vi "TDC_Prototype.vi"() -> ()   [LabVIEW 2025]
uses:
  Desktop/STM-Auto-Project/QMH CTLS/Scan_Params (QMH).ctl
  TDC_SubVI/TEMP_SWEEPER.ctl
  Downloads/OneDrive_2025-09-03/Instrument Controls/Temp Cntrl.ctl
  Desktop/Magnetic Drift Correction/XY_Coords(Final).ctl
panel:
  out "Z-Controller on/off status":bool
  in  "Field and Temp Range":T1={"VISA (Magnet)"="COM4", "Fields(T)"=[], "Temps(K)"=[], "VISA (Temp) "="COM1"}
  out "error out":errorcluster
  in  "Serial Configuration":T2={"Baud Rate"=57600, "Parity"=1, "Data Bits"=7, "Stop Bits"=10, "Flow Control"=0}
  out "Current Index":i32
  out "Translation (m)":T3
  out "Final coordinates (m)":cluster{"Xc":sgl, "Yc":sgl} {"Yc" format="%.4p"; "Xc" format="%.4p"}
  out "Initial coordinates (m)":cluster{"Xc":sgl, "Yc":sgl} {"Yc" format="%.4p"; "Xc" format="%.4p"}
  in  "stop":bool
  in  "Start":bool
  # "Main goals,\n\nSet base line: Do initial bias and scan\n\nChange temp: Init temp, temp on, temp stab,\n\nInter scan, move frame, final scan, bias shit,\n\nNext temp? Prep next field though reinialization, determine if higher range is needed, apply field by changing setpoint\n\nInter scan, move frame, final scan, bias shit,"
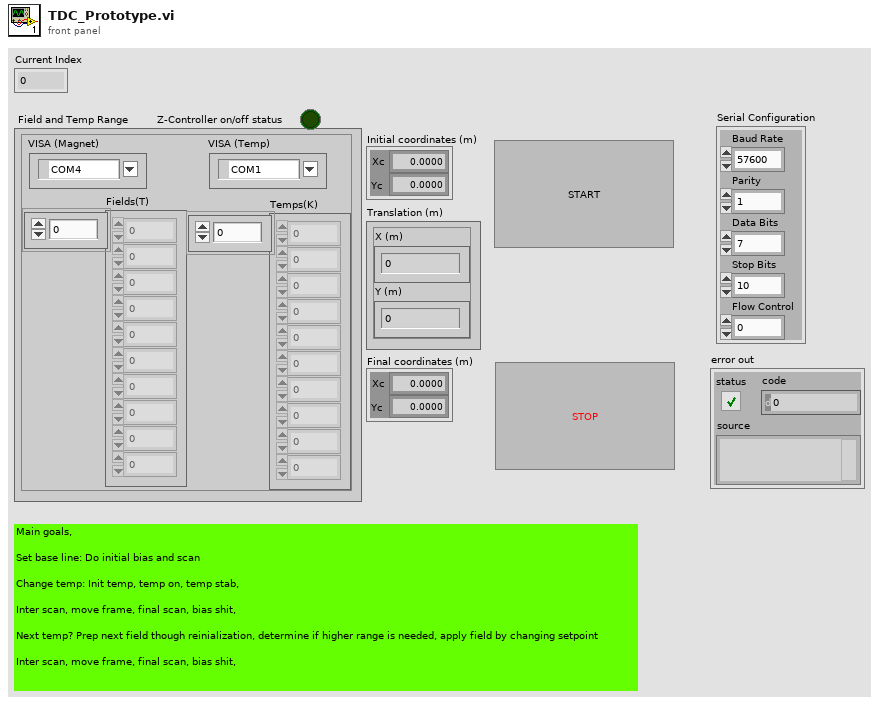
[diagram p1: front panel]
types:
  T1 = cluster{"VISA (Magnet)":refnum<visa-resource-name>, "Fields(T)":dbl[], "Temps(K)":dbl[], "VISA (Temp) ":refnum<visa-resource-name>}
  T2 = cluster{"Baud Rate":u32, "Parity":u16, "Data Bits":u16, "Stop Bits":u16, "Flow Control":u16}
  T3 = typedef "XY_Coords(Final).ctl" = cluster{"X (m)":dbl, "Y (m)":dbl}
  T4 = enum16{"1. BIAS", "2. INIT_SCAN", "3. SCAN_IDLE", "4. INTER_SCAN", "5. NEW_COORDS_&_FRAME", "6. FINAL_SCAN", "7. POLL BIAS ", "8. Z-CONT.", "9. STOP"}
  T5 = enum16{"SET TEMP", "SWEEP IDLE", "NEXT TEMP", "SWEEP DONE"}
  T6 = enum16{"1. INIT TEMP", "2. TC ON", "3. POLL_TEMPS", "4. TEMP_STAB", "5. TC IDLE", "6. APPLY NEXT TEMP", "7. TC OFF (Reset)"}
  T7 = typedef "Temp Cntrl.ctl" = cluster{"Range (0:Off)":u16, "Manual Output (0.00 %)":dbl, "Rate (D) (0.0 %)":dbl, "Reset (I) (20.0)":dbl, "Gain (P) (50.0)":dbl, "Power Up Enable (F: Disable)":bool, "Max User Current (2.000)":dbl, "Heater Resistance (1:25 Ohms)":u16, "Max Current (0:User Specified)":u16, "Heater Out Display (1:Current)":u16, "Mode (0:Off)":u16, "Input (0:None)":u16, "Target Temp (K)":dbl, "Serial Configuration":cluster{"Baud Rate":u32, "Parity":u16, "Data Bits":u16, "Stop Bits":u16, "Flow Control":u16}, "VISA resource name":refnum<visa-resource-name>, "Configure Control Parameters (0: Configure)":u16, "Enable Setpoint (F:Disable)":bool, "Input (0:A)":u16, "Data Source (0:Kelvin)":u16, "Output's Control Loop (1:1)":u16, "STND DEV Threshold ":dbl, "Mean Tolerance ":dbl, "Current State":enum16{"1. INIT TEMP", "2. TC ON", "3. POLL_TEMPS", "4. TEMP_STAB", "5. TC IDLE", "6. APPLY NEXT TEMP", "7. TC OFF (Reset)"}}
  T8 = typedef "TEMP_SWEEPER.ctl" = cluster{"Temps(K)":dbl[], "Sweep States":enum16{"SET TEMP", "SWEEP IDLE", "NEXT TEMP", "SWEEP DONE"}}
  T9 = typedef "Scan_Params (QMH).ctl" = cluster{"Setpoint (I)":dbl[], "Bias (V)":dbl[], "Number of scans":u8, "Port number (3364)":u32, "Avoid zero threshold (V)":dbl, "Current State":enum16{"1. BIAS", "2. INIT_SCAN", "3. SCAN_IDLE", "4. INTER_SCAN", "5. NEW_COORDS_&_FRAME", "6. FINAL_SCAN", "7. POLL BIAS ", "8. Z-CONT.", "9. STOP"}}
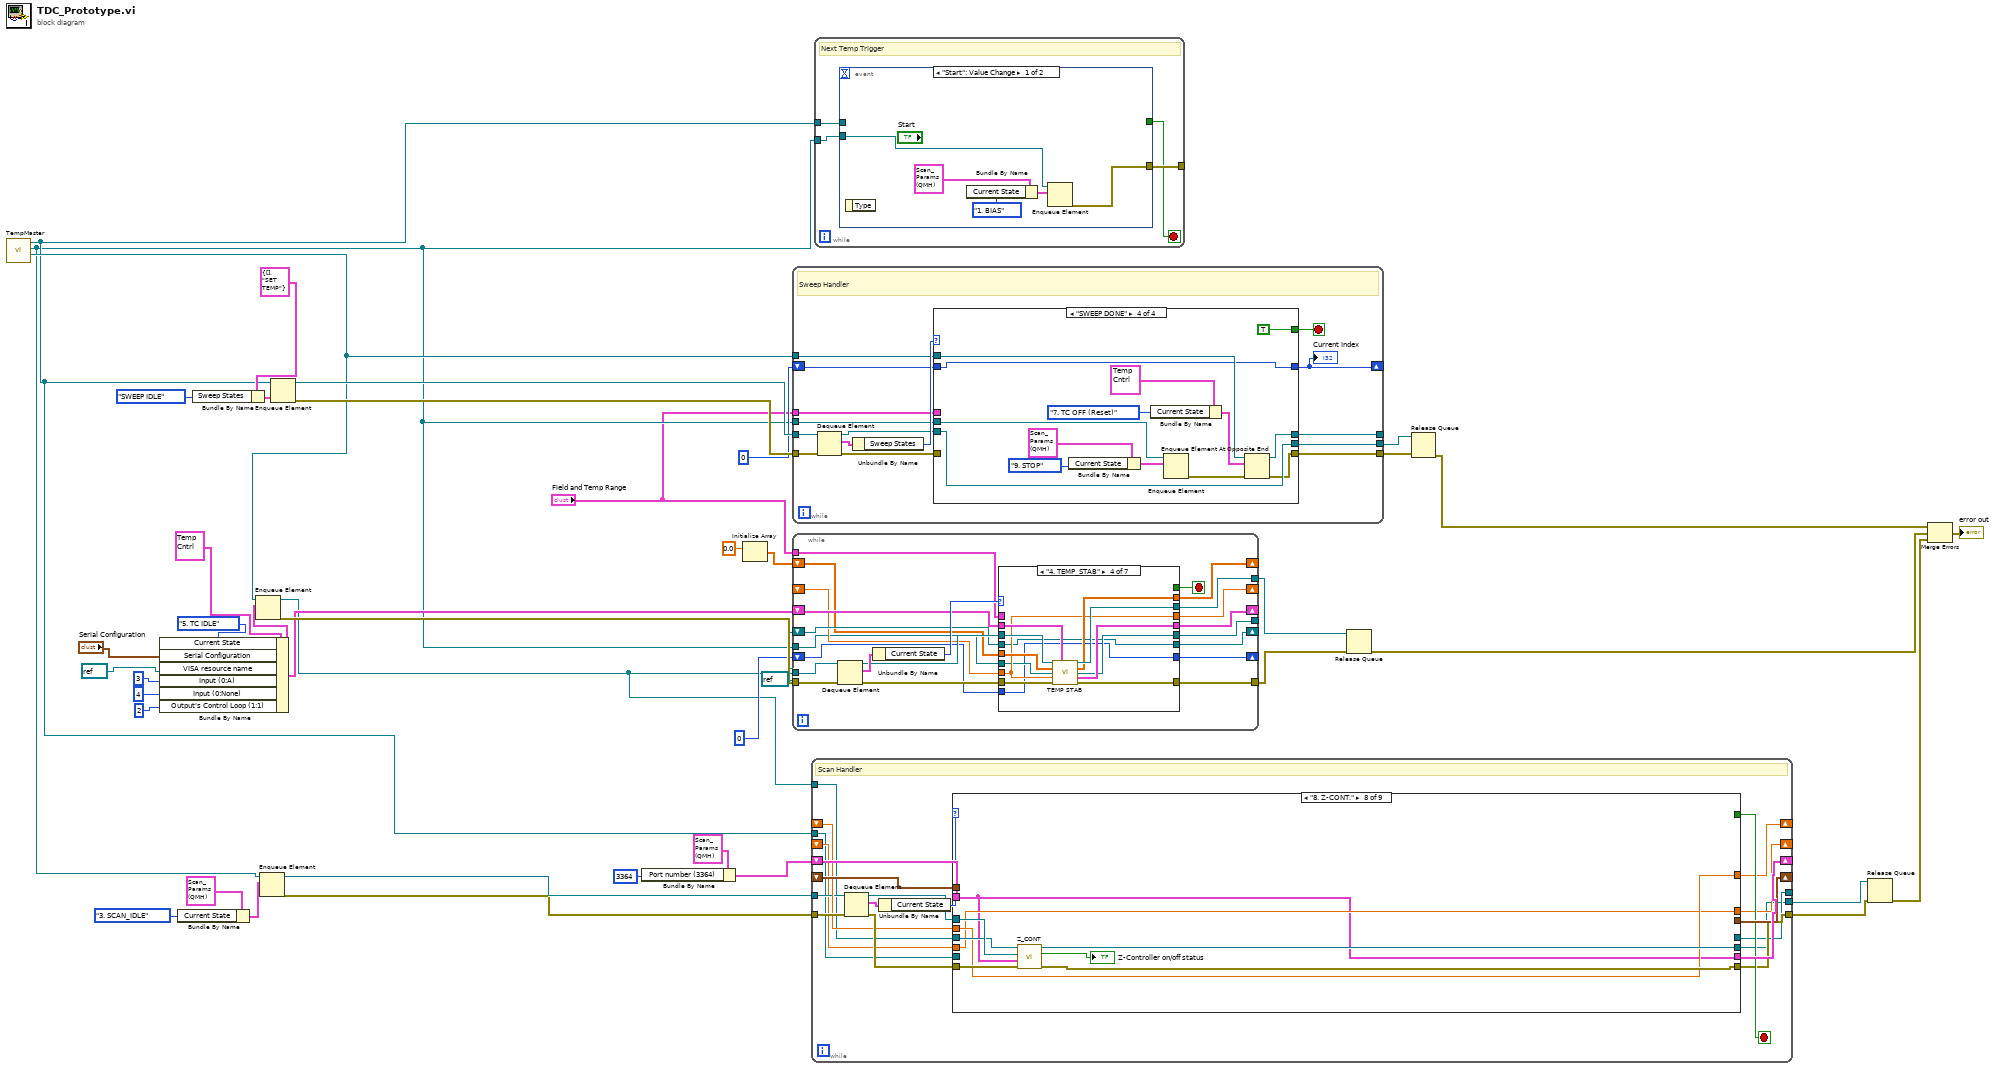
[diagram p0: block diagram]
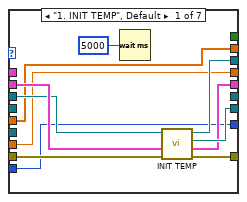
[diagram p2: hidden frame]
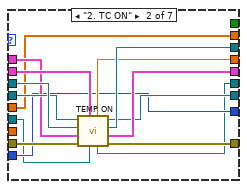
[diagram p3: hidden frame]
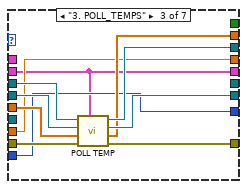
[diagram p4: hidden frame]
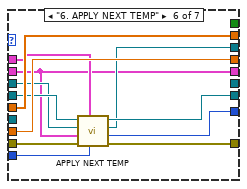
[diagram p6: hidden frame]
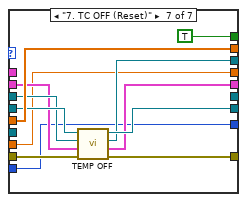
[diagram p7: hidden frame]
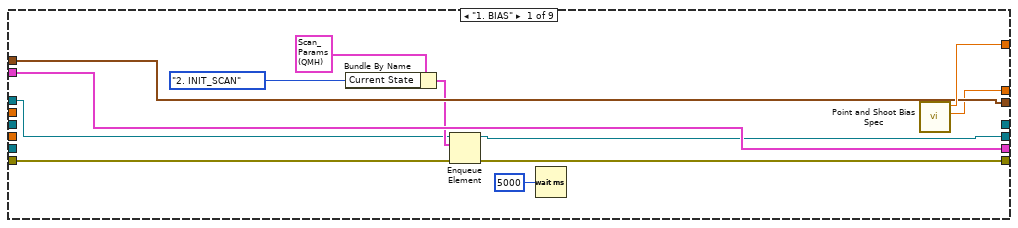
[diagram p8: hidden frame]
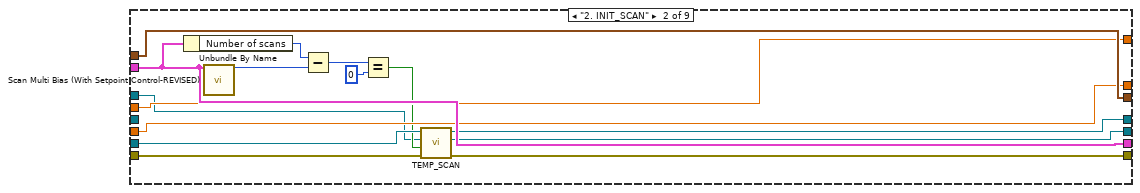
[diagram p9: hidden frame]
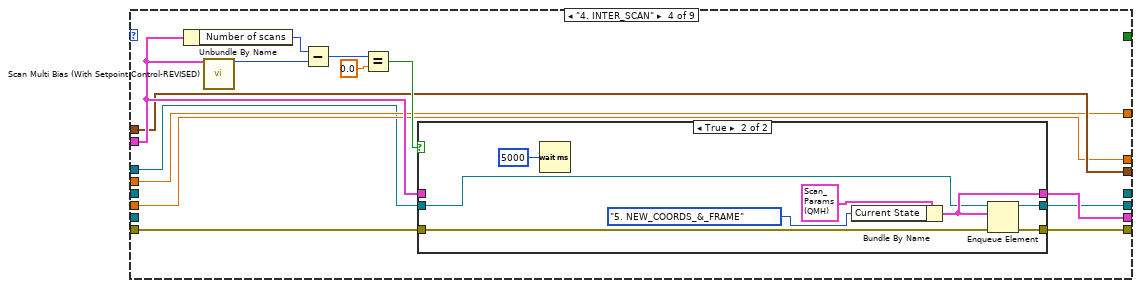
[diagram p11: hidden frame]
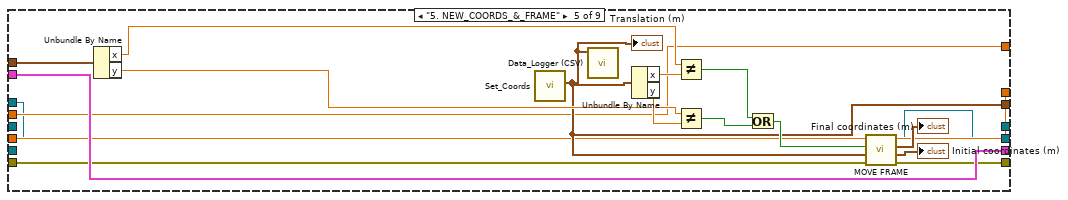
[diagram p13: hidden frame]
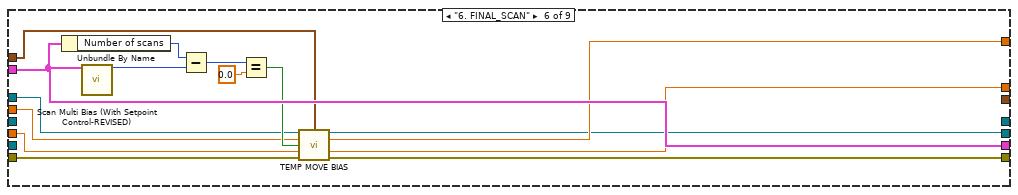
[diagram p14: hidden frame]
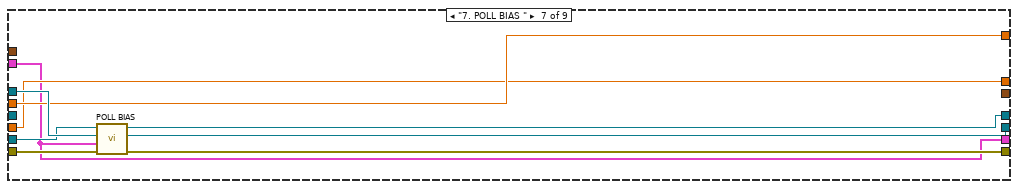
[diagram p15: hidden frame]
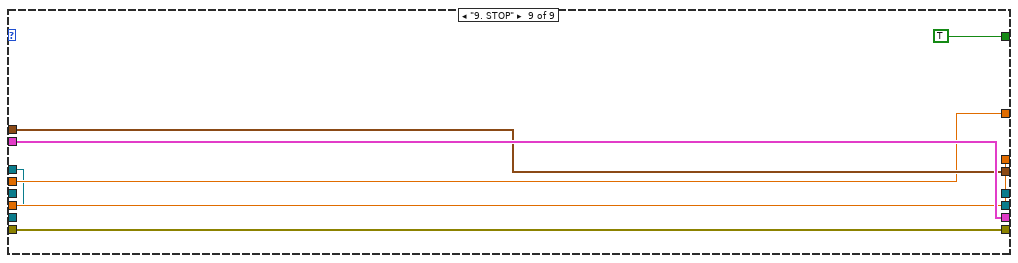
[diagram p16: hidden frame]
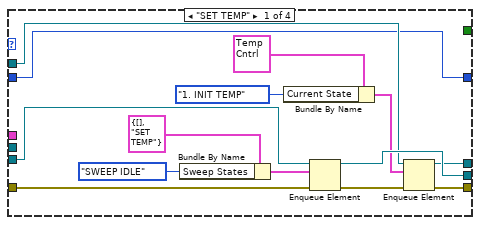
[diagram p17: hidden frame]
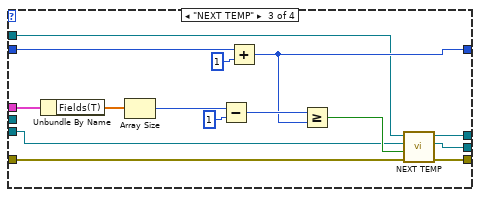
[diagram p19: hidden frame]
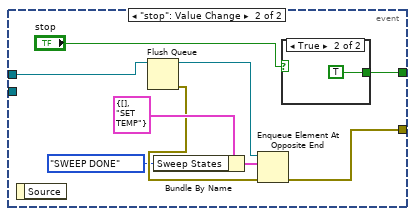
[diagram p20: hidden frame]
diagram:
  n1 = call "TempMaster.vi"() -> ("TempQ"=w27:refnum<queue>, "ScanQ"=w12:refnum<queue>, "SweepQ"=w17:refnum<queue>)  [unwired: 9 in]
  n2 = Bundle By Name(cluster=T7 {"Range (0:Off)"=0, "Manual Output (0.00 %)"=0.0, "Rate (D) (0.0 %)"=0.0, "Reset (I) (20.0)"=20.0, "Gain (P) (50.0)"=50.0, "Power Up Enable (F: Disable)"=FALSE, "Max User Current (2.000)"=2.0, "Heater Resistance (1:25 Ohms)"=1, "Max Current (0:User Specified)"=0, "Heater Out Display (1:Current)"=1, "Mode (0:Off)"=1, "Input (0:None)"=4, "Target Temp (K)"=5.0, "Serial Configuration"={"Baud Rate"=57600, "Parity"=1, "Data Bits"=7, "Stop Bits"=10, "Flow Control"=0}, "VISA resource name"="", "Configure Control Parameters (0: Configure)"=0, "Enable Setpoint (F:Disable)"=FALSE, "Input (0:A)"=3, "Data Source (0:Kelvin)"=0, "Output's Control Loop (1:1)"=2, "STND DEV Threshold "=0.1, "Mean Tolerance "=0.02, "Current State"=enum."1. INIT TEMP"} ("element"), "Current State"=T6."5. TC IDLE", "Serial Configuration"="Serial Configuration", "VISA resource name"=refnum<visa-resource-name> refnum, "Input (0:A)"=u16 3, "Input (0:None)"=u16 4, "Output's Control Loop (1:1)"=u16 2) -> (w22:T7)
  n3 = Bundle By Name(cluster=T9 {"Setpoint (I)"=[], "Bias (V)"=[], "Number of scans"=1, "Port number (3364)"=3364, "Avoid zero threshold (V)"=0.004999999888241291, "Current State"=enum."1. BIAS"} ("element"), "Current State"=T4."3. SCAN_IDLE") -> (w37:T9)
  n4 = Bundle By Name(cluster=T8 {"Temps(K)"=[], "Sweep States"=enum."SET TEMP"} ("Temp and Field Range"), "Sweep States"=T5."SWEEP IDLE") -> (w41:T8)
  n5 = Enqueue Element(queue=w27, element=w22) -> (queue out=w1:refnum<queue>, error out=w28:errorcluster)  [unwired: 2 in, 1 out]
  n6 = Enqueue Element(queue=w12, element=w37) -> (queue out=w39:refnum<queue>, error out=w38:errorcluster)  [unwired: 2 in, 1 out]
  n7 = Enqueue Element(queue=w17, element=w41) -> (queue out=w42:refnum<queue>, error out=w40:errorcluster)  [unwired: 2 in, 1 out]
  n8 = Bundle By Name(cluster=T9 {"Setpoint (I)"=[], "Bias (V)"=[], "Number of scans"=1, "Port number (3364)"=3364, "Avoid zero threshold (V)"=0.004999999888241291, "Current State"=enum."1. BIAS"} ("element"), "Port number (3364)"=u32 3364) -> (w34:T9)
  n9 = Initialize Array(0.0 ("element")) -> (w18:dbl[])  [unwired: 1 in]
  n10 = while {
    tunnel: w42 -> [w57]
    shift-right: [w50] -> _
    shift-left: 0 ("Current Index") -> [w51]
    tunnel: w27 -> [w49]
    tunnel: w40 -> [w56]
    tunnel: "Field and Temp Range" -> [w52]
    tunnel: [w48] -> w9
    tunnel: [w47] -> _
    tunnel: [w46] -> w8
    tunnel: w12 -> [w44]
    stop <- w43 stop-if-true
    # "Sweep Handler"
    n11 = Dequeue Element(queue=w57, error in (no error)=w56) -> (queue out=w53:refnum<queue>, element=w55:T8, error out=w45:errorcluster)  [unwired: 1 in, 1 out]
    n12 = Unbundle By Name(w55) -> ("Sweep States"=w54:T5)
    n13 = case shown="\"SWEEP DONE\"" w54 {
      tunnel: w53 -> [w71 w73 w80 w96]
      tunnel: w52 -> [_ _ w86 _]
      tunnel: w51 -> [w60 w75 w84 w94]
      tunnel: [w60 w75 w83 w94] -> w50
      tunnel: w49 -> [w63 w74 w81 w103]
      tunnel: [w66 w73 w76 w96] -> w48
      tunnel: [w62 w74 w77 w97] -> w47
      tunnel: [w61 w72 w79 w95] -> w46
      tunnel: w45 -> [w68 w72 w78 _]
      tunnel: w44 -> [_ _ _ w101]
      tunnel: [_ _ _ TRUE] -> w43
      frame "SET TEMP" {
        n14 = Bundle By Name(cluster=T8 {"Temps(K)"=[], "Sweep States"=enum."SET TEMP"} ("Temp and Field Range"), "Sweep States"=T5."SWEEP IDLE") -> (w69:T8)
        n15 = Bundle By Name(cluster=T7 {"Range (0:Off)"=0, "Manual Output (0.00 %)"=0.0, "Rate (D) (0.0 %)"=0.0, "Reset (I) (20.0)"=20.0, "Gain (P) (50.0)"=50.0, "Power Up Enable (F: Disable)"=FALSE, "Max User Current (2.000)"=2.0, "Heater Resistance (1:25 Ohms)"=1, "Max Current (0:User Specified)"=0, "Heater Out Display (1:Current)"=1, "Mode (0:Off)"=1, "Input (0:None)"=4, "Target Temp (K)"=5.0, "Serial Configuration"={"Baud Rate"=57600, "Parity"=1, "Data Bits"=7, "Stop Bits"=10, "Flow Control"=0}, "VISA resource name"="", "Configure Control Parameters (0: Configure)"=0, "Enable Setpoint (F:Disable)"=FALSE, "Input (0:A)"=3, "Data Source (0:Kelvin)"=0, "Output's Control Loop (1:1)"=2, "STND DEV Threshold "=0.1, "Mean Tolerance "=0.02, "Current State"=enum."1. INIT TEMP"} ("element"), "Current State"=T6."1. INIT TEMP") -> (w64:T7)
        n16 = Enqueue Element(queue=w71, element=w69, error in (no error)=w68) -> (queue out=w66:refnum<queue>, error out=w67:errorcluster)  [unwired: 1 in, 1 out]
        n17 = Enqueue Element(queue=w63, element=w64, error in (no error)=w67) -> (queue out=w62:refnum<queue>, error out=w61:errorcluster)  [unwired: 1 in, 1 out]
      }
      frame "SWEEP IDLE" {
      }
      frame "NEXT TEMP" {
        n18 = Unbundle By Name(w86) -> ("Fields(T)"=w85:dbl[])
        n19 = Array Size(array=w85) -> (size(s)=w89:i32)
        n20 = Subtract(x=w89, y=1) -> (x-y=w87:i32)
        n21 = Add(x=w84, y=1) -> (x+y=w83:i32)
        n22 = Greater Or Equal?(x=w87, y=w83) -> (x >= y?=w82:bool)
        n23 = call "NEXT TEMP.vi"("error in (no error)"=w78, "Boolean"=w82, "SweepQ"=w80, "TempQ"=w81) -> ("error out"=w79:errorcluster, "SweepQ Out"=w76:refnum<queue>, "TEMPQ Out"=w77:refnum<queue>)  [unwired: 5 in]
      }
      frame "SWEEP DONE" {
        n24 = Bundle By Name(cluster=T9 {"Setpoint (I)"=[], "Bias (V)"=[], "Number of scans"=1, "Port number (3364)"=3364, "Avoid zero threshold (V)"=0.004999999888241291, "Current State"=enum."1. BIAS"} ("element"), "Current State"=T4."9. STOP") -> (w100:T9)
        n25 = Bundle By Name(cluster=T7 {"Range (0:Off)"=0, "Manual Output (0.00 %)"=0.0, "Rate (D) (0.0 %)"=0.0, "Reset (I) (20.0)"=20.0, "Gain (P) (50.0)"=50.0, "Power Up Enable (F: Disable)"=FALSE, "Max User Current (2.000)"=2.0, "Heater Resistance (1:25 Ohms)"=1, "Max Current (0:User Specified)"=0, "Heater Out Display (1:Current)"=1, "Mode (0:Off)"=1, "Input (0:None)"=4, "Target Temp (K)"=5.0, "Serial Configuration"={"Baud Rate"=57600, "Parity"=1, "Data Bits"=7, "Stop Bits"=10, "Flow Control"=0}, "VISA resource name"="", "Configure Control Parameters (0: Configure)"=0, "Enable Setpoint (F:Disable)"=FALSE, "Input (0:A)"=3, "Data Source (0:Kelvin)"=0, "Output's Control Loop (1:1)"=2, "STND DEV Threshold "=0.1, "Mean Tolerance "=0.02, "Current State"=enum."1. INIT TEMP"} ("element"), "Current State"=T6."7. TC OFF (Reset)") -> (w98:T7)
        n26 = Enqueue Element(queue=w101, element=w100) -> (error out=w104:errorcluster)  [unwired: 2 in, 2 out]
        n27 = Enqueue Element At Opposite End(queue=w103, element=w98, error in (no error)=w104) -> (queue out=w97:refnum<queue>, error out=w95:errorcluster)  [unwired: 1 in, 1 out]
      }
    }
    "Current Index" <- w50
  }
  n28 = while {
    tunnel: w1 -> [w126]
    tunnel: w28 -> [w125]
    shift-right: [w115] -> _
    shift-left: w22 -> [w122]
    tunnel: "Field and Temp Range" -> [w120]
    shift-right: [w119] -> _
    shift-left: refnum<visa-resource-name> refnum ("VISA resource name out") -> [w114]
    tunnel: [w118] -> w10
    tunnel: [w116] -> w11
    shift-right: [w110] -> _
    shift-left: _ -> [w113]
    shift-right: [w111] -> _
    shift-left: w18 -> [w112]
    tunnel: w12 -> [w109]
    tunnel: [w108] -> _
    shift-right: [w106] -> _
    shift-left: 0 -> [w107]
    stop <- w105 stop-if-true
    n29 = Dequeue Element(queue=w126, error in (no error)=w125) -> (queue out=w117:refnum<queue>, element=w124:T7, error out=w121:errorcluster)  [unwired: 1 in, 1 out]
    n30 = Unbundle By Name(w124) -> ("Current State"=w123:T6)
    n31 = case shown="\"4. TEMP_STAB\"" w123 {
      tunnel: w122 -> [w137 w151 w152 w173 w177 w183 w201]
      tunnel: w121 -> [w136 w145 w161 w172 w178 w189 w204]
      tunnel: w120 -> [_ w144 _ _ _ w184 _]
      tunnel: [w135 w143 w160 w163 w179 w188 w203] -> w119
      tunnel: [w132 w148 w157 w170 w178 w185 w200] -> w118
      tunnel: w117 -> [w134 w150 w159 w174 w180 w187 w202]
      tunnel: [w133 w149 w158 w171 w180 w186 w199] -> w116
      tunnel: [w130 w147 w152 w167 w177 w183 w198] -> w115
      tunnel: w114 -> [_ w146 w162 w163 w179 w190 w205]
      tunnel: [w128 w142 w154 w168 w181 w193 w196] -> w110
      tunnel: w113 -> [w128 _ w154 w168 w181 w193 w196]
      tunnel: w112 -> [w129 w141 w156 w175 w182 w194 w206]
      tunnel: [w129 w141 w155 w169 w182 w194 w206] -> w111
      tunnel: w109 -> [_ w139 _ w166 _ _ _]
      tunnel: [_ w138 _ w165 _ _ _] -> w108
      tunnel: w107 -> [w127 w140 w153 w164 w176 w192 w197]
      tunnel: [w127 w140 w153 w164 w176 w191 w197] -> w106
      tunnel: [_ _ _ _ _ _ TRUE] -> w105
      frame "1. INIT TEMP", Default {
        n32 = Wait (ms)(milliseconds to wait=u32 5000) -> ()  [unwired: 1 out]
        n33 = call "INIT TEMP.vi"("error in (no error)"=w136, "element"=w137, "Queue in"=w134) -> ("error out"=w132:errorcluster, "output cluster"=w130:T7, "VISA resource name out"=w135:refnum<visa-resource-name>, "Queue out"=w133:refnum<queue>)  [unwired: 5 in]
      }
      frame "2. TC ON" {
        n34 = call "TEMP ON.vi"("ScanQ in"=w139, "element in"=w151, "error in (no error)"=w145, "Field and Temp Range"=w144, "TempQ in"=w150, "VISA Refnum in"=w146) -> ("error out"=w148:errorcluster, "element out"=w147:T7, "TempQ out"=w149:refnum<queue>, "VISA Refnum out"=w143:refnum<visa-resource-name>, "ScanQ out"=w138:refnum<queue>, "Setpoint"=w142:dbl)
      }
      frame "3. POLL_TEMPS" {
        n35 = call "POLL TEMP.vi"("element"=w152, "error in (no error)"=w161, "Array in"=w156, "VISA resource name in"=w162, "Queue in"=w159) -> ("error out"=w157:errorcluster, "Array"=w155:dbl[], "VISA resource name out"=w160:refnum<visa-resource-name>, "Queue out"=w158:refnum<queue>)  [unwired: 3 in]
      }
      frame "4. TEMP_STAB" {
        n36 = call "TEMP STAB.vi"("Queue in"=w174, "element in"=w173, "Array in"=w175, "ScanQ In"=w166, "Setpoint"=w168, "error in (no error)"=w172) -> ("Queue out"=w171:refnum<queue>, "Array out"=w169:dbl[], "ScanQ"=w165:refnum<queue>, "element out"=w167:T7, "error out"=w170:errorcluster)  [unwired: 5 in]
      }
      frame "5. TC IDLE" {
      }
      frame "6. APPLY NEXT TEMP" {
        n37 = call "APPLY NEXT TEMP.vi"("Numeric in"=w192, "Field and Temp Range"=w184, "error in (no error)"=w189, "element in"=w183, "TempQ in"=w187, "VISA Refnum in"=w190) -> ("error out"=w185:errorcluster, "Numeric out"=w191:i32, "TempQ out"=w186:refnum<queue>, "VISA Refnum out"=w188:refnum<visa-resource-name>)  [unwired: 2 in]
      }
      frame "7. TC OFF (Reset)" {
        n38 = call "TEMP OFF.vi"("error in (no error)"=w204, "element in"=w201, "TempQ in"=w202, "VISA Refnum in"=w205) -> ("error out"=w200:errorcluster, "element out"=w198:T7, "TempQ out"=w199:refnum<queue>, "VISA Refnum out"=w203:refnum<visa-resource-name>)  [unwired: 4 in]
      }
    }
  }
  n39 = while {
    tunnel: w38 -> [w220]
    shift-right: [w225] -> _
    shift-left: w34 -> [w226]
    shift-right: [w224] -> _
    shift-left: _ -> [w223]
    tunnel: [w221] -> w36
    tunnel: [w218] -> _
    shift-right: [w216] -> _
    shift-left: _ -> [w217]
    tunnel: w39 -> [w215]
    shift-right: [w212] -> _
    shift-left: _ -> [w211]
    tunnel: w17 -> [w210]
    tunnel: [w209] -> w16
    tunnel: w1 -> [w207]
    stop <- w222 stop-if-true
    # "Scan Handler"
    n40 = Dequeue Element(queue=w215, error in (no error)=w220) -> (queue out=w208:refnum<queue>, element=w213:T9, error out=w219:errorcluster)  [unwired: 1 in, 1 out]
    n41 = Unbundle By Name(w213) -> ("Current State"=w214:T4)
    n42 = case shown="\"8. Z-CONT.\"" w214 {
      tunnel: w226 -> [w237 w250 w257 w266 w301 w313 w317 w326 w339]
      tunnel: w219 -> [w233 w243 _ w263 w291 w310 w325 w330 w340]
      tunnel: [w237 w250 w257 w267 w301 w313 w317 w326 w339] -> w225
      tunnel: [w236 w248 w258 w265 w288 _ _ _ w338] -> w224
      tunnel: w223 -> [w236 w248 w258 w265 w293 w308 _ _ w338]
      tunnel: [_ _ _ _ _ _ _ _ TRUE] -> w222
      tunnel: [w234 w239 _ w264 w292 w309 w320 w331 w340] -> w221
      tunnel: [_ w242 _ _ _ _ w321 _ _] -> w218
      tunnel: w217 -> [_ w247 w256 w262 w287 w306 w319 w328 w337]
      tunnel: [w238 w247 w256 w262 w287 w304 w319 w328 w337] -> w216
      tunnel: [w230 w246 w255 w261 w286 w303 w318 w327 w336] -> w212
      tunnel: w211 -> [_ w246 w255 w261 w286 w305 w318 w327 w336]
      tunnel: w210 -> [_ w245 _ _ _ _ w322 _ _]
      tunnel: [w228 w241 w254 w259 w284 w302 w323 w332 w335] -> w209
      tunnel: w208 -> [w229 w240 w254 w260 w285 w307 w324 w333 w335]
      tunnel: w207 -> [_ _ _ _ _ _ _ w329 _]
      frame "1. BIAS" {
        n43 = Bundle By Name(cluster=T9 {"Setpoint (I)"=[], "Bias (V)"=[], "Number of scans"=1, "Port number (3364)"=3364, "Avoid zero threshold (V)"=0.004999999888241291, "Current State"=enum."1. BIAS"} ("element"), "Current State"=T4."2. INIT_SCAN") -> (w231:T9)
        n44 = Enqueue Element(queue=w229, element=w231, error in (no error)=w233) -> (queue out=w228:refnum<queue>, error out=w234:errorcluster)  [unwired: 1 in, 1 out]
        n45 = Wait (ms)(milliseconds to wait=u32 5000) -> ()  [unwired: 1 out]
        n46 = call "Point and Shoot Bias Spec.vi"() -> ("Initial Y (m)"=w230:dbl, "Inital X (m)"=w238:dbl)  [unwired: 10 in]
      }
      frame "2. INIT_SCAN" {
        n47 = Unbundle By Name(w250) -> ("Number of scans"=w249:u8)
        n48 = call "Scan Multi Bias (With Setpoint Control-REVISED).vi"("Scan Parameters"=w250) -> ("Scan"=w251:u8)  [unwired: 13 in, 1 out]
        n49 = Subtract(x=w249, y=w251) -> (x-y=w253:u8)
        n50 = Equal?(x=w253, y=u8 0) -> (x = y?=w244:bool)
        n51 = call "TEMP_SCAN.vi"("error in (no error)"=w243, "Boolean"=w244, "ScanQ in"=w240, "SweepQ in"=w245) -> ("error out"=w239:errorcluster, "ScanQ out"=w241:refnum<queue>, "SweepQ out"=w242:refnum<queue>)  [unwired: 5 in]
      }
      frame "3. SCAN_IDLE" {
      }
      frame "4. INTER_SCAN" {
        n52 = Unbundle By Name(w266) -> ("Number of scans"=w268:u8)
        n53 = call "Scan Multi Bias (With Setpoint Control-REVISED).vi"("Scan Parameters"=w266) -> ("Scan"=w269:u8)  [unwired: 13 in, 1 out]
        n54 = Subtract(x=w268, y=w269) -> (x-y=w271:u8)
        n55 = Equal?(x=w271, y=0.0) -> (x = y?=w270:bool)
        n56 = case shown="True" w270 {
          tunnel: [w275 w279] -> w267
          tunnel: w266 -> [w275 _]
          tunnel: [w274 w282] -> w264
          tunnel: w263 -> [w274 w281]
          tunnel: w260 -> [w273 w278]
          tunnel: [w273 w277] -> w259
          frame False {
          }
          frame True {
            n57 = Wait (ms)(milliseconds to wait=u32 5000) -> ()  [unwired: 1 out]
            n58 = Bundle By Name(cluster=T9 {"Setpoint (I)"=[], "Bias (V)"=[], "Number of scans"=1, "Port number (3364)"=3364, "Avoid zero threshold (V)"=0.004999999888241291, "Current State"=enum."2. INIT_SCAN"} ("element"), "Current State"=T4."5. NEW_COORDS_&_FRAME") -> (w279:T9)
            n59 = Enqueue Element(queue=w278, element=w279, error in (no error)=w281) -> (queue out=w277:refnum<queue>, error out=w282:errorcluster)  [unwired: 1 in, 1 out]
          }
        }
      }
      frame "5. NEW_COORDS_&_FRAME" {
        n60 = Unbundle By Name(w293) -> ("x"=w295:dbl, "y"=w294:dbl)
        n61 = call "Set_Coords.vi"() -> ("return value"=w288:cluster{"x":dbl, "y":dbl})  [unwired: 10 in, 1 out]
        "Translation (m)" <- w288
        n62 = call "Data_Logger (CSV).vi"("Translation (m)"=w288) -> ()  [unwired: 11 in]
        n63 = Unbundle By Name(w288) -> ("x"=w298:dbl, "y"=w297:dbl)
        n64 = Not Equal?(x=w295, y=w298) -> (x != y?=w300:bool)
        n65 = Not Equal?(x=w294, y=w297) -> (x != y?=w299:bool)
        n66 = Or(x=w300, y=w299) -> (x .or. y?=w296:bool)
        n67 = call "MOVE FRAME.vi"("error in (no error)"=w291, "return value"=w288, "Boolean"=w296, "Queue in"=w285) -> ("error out"=w292:errorcluster, "Initial coordinates (m)"=→"Initial coordinates (m)":cluster{"Xc":sgl, "Yc":sgl}, "Final coordinates (m)"=→"Final coordinates (m)":cluster{"Xc":sgl, "Yc":sgl}, "Queue out"=w284:refnum<queue>)  [unwired: 4 in]
      }
      frame "6. FINAL_SCAN" {
        n68 = Unbundle By Name(w313) -> ("Number of scans"=w312:u8)
        n69 = call "Scan Multi Bias (With Setpoint Control-REVISED).vi"("Scan Parameters"=w313) -> ("Scan"=w314:u8)  [unwired: 13 in, 1 out]
        n70 = Subtract(x=w312, y=w314) -> (x-y=w315:u8)
        n71 = Equal?(x=w315, y=0.0) -> (x = y?=w311:bool)
        n72 = call "TEMP MOVE BIAS.vi"("ScanQ in"=w307, "Translation"=w308, "x"=w306, "Boolean"=w311, "y"=w305, "error in (no error)"=w310) -> ("ScanQ out"=w302:refnum<queue>, "X (m)"=w304:sgl, "Y (m)"=w303:sgl, "error out"=w309:errorcluster)  [unwired: 6 in]
      }
      frame "7. POLL BIAS " {
        n73 = call "POLL BIAS.vi"("error in (no error)"=w325, "element"=w317, "ScanQ in"=w324, "Queue in"=w322) -> ("error out"=w320:errorcluster, "ScanQ out"=w323:refnum<queue>, "Queue out"=w321:refnum<queue>)  [unwired: 5 in]
      }
      frame "8. Z-CONT." {
        n74 = call "Z_CONT.vi"("error in (no error)"=w330, "element"=w326, "ScanQ in"=w333, "Queue in"=w329) -> ("error out"=w331:errorcluster, "Z-Controller on/off status"=→"Z-Controller on/off status":bool, "Queue out"=w332:refnum<queue>)  [unwired: 5 in]
      }
      frame "9. STOP" {
      }
    }
  }
  n75 = while {
    tunnel: [w345] -> _
    tunnel: w17 -> [w343]
    tunnel: w12 -> [w342]
    stop <- w344 stop-if-true
    # "Next Temp Trigger"
    n76 = event shown="[0] \"Start\": Value Change" {
      selector: _ -> [_ _]
      dyn-events: _ -> [_ _]
      timeout: _ -> [_ _]
      tunnel: [w350 w359] -> w345
      tunnel: [_ w357] -> w344
      tunnel: w343 -> [_ w354]
      tunnel: w342 -> [w348 _]
      event "Start": Value Change {
        n77 = event-data() -> ()  [unwired: 1 in, 1 out]
        n78 = Bundle By Name(cluster=T9 {"Setpoint (I)"=[], "Bias (V)"=[], "Number of scans"=1, "Port number (3364)"=3364, "Avoid zero threshold (V)"=0.004999999888241291, "Current State"=enum."1. BIAS"} ("element"), "Current State"=T4."1. BIAS") -> (w347:T9)
        n79 = Enqueue Element(queue=w348, element=w347) -> (error out=w350:errorcluster)  [unwired: 2 in, 2 out]
      }
      event "stop": Value Change {
        n80 = event-data() -> ()  [unwired: 1 in, 1 out]
        n81 = Flush Queue(queue=w354) -> (queue out=w353:refnum<queue>, error out=w352:errorcluster)  [unwired: 1 in, 1 out]
        n82 = Bundle By Name(cluster=T8 {"Temps(K)"=[], "Sweep States"=enum."SET TEMP"} ("Temp and Field Range"), "Sweep States"=T5."SWEEP DONE") -> (w355:T8)
        n83 = Enqueue Element At Opposite End(queue=w353, element=w355, error in (no error)=w352) -> (error out=w359:errorcluster)  [unwired: 1 in, 2 out]
        n84 = case shown="True" "stop" {
          tunnel: [FALSE ("stop 2") TRUE ("stop 2")] -> w357
          frame False {
          }
          frame True {
          }
        }
      }
    }
  }
  n85 = Release Queue(queue=w11, error in (no error)=w10) -> (error out=w6:errorcluster)  [unwired: 1 in, 2 out]
  n86 = Release Queue(queue=w9, error in (no error)=w8) -> (error out=w7:errorcluster)  [unwired: 1 in, 2 out]
  n87 = Release Queue(queue=w16, error in (no error)=w36) -> (error out=w5:errorcluster)  [unwired: 1 in, 2 out]
  n88 = Merge Errors(w7, w6, w5) -> (→"error out":errorcluster)
